vi "init.vi"(8 "error in":errorcluster, 10 "TBM module configuration in":refnum<class "TBM module configuration.lvclass">, 11 "Engine to Engine Communication runtime in":refnum<class "E2E Runtime (RT FIFO).lvclass">) -> (0 "error out":errorcluster, 1 "data allocations":T1, 2 "execution settings":T4, 3 "Engine to Engine Communication runtime out":refnum<class "E2E Runtime (RT FIFO).lvclass">)   [LabVIEW 2015, in "E2E Runtime (RT FIFO).lvclass"]
doc: "Provides an interface for initializing a module at runtime. While this interface performs no operations, a child should provide an override which may open any necessary references or sessions, allocate necessary memory, and perform any final configuration validataion before providing the full configuration <b>execution data</b> to the calling process."
uses:
  E2E Runtime (RT FIFO).lvclass
  <vilib>/NI/Tag Bus Module Framework/module configuration/TBM module configuration.lvclass
  <vilib>/NI/Tag Bus Module Framework/runtime/execution settings.ctl
  <vilib>/NI/Tag Bus Module Framework/channel/data tables.ctl
  <vilib>/NI/Tag Bus/dictionary/data dictionary.lvclass
  <vilib>/NI/Tag Bus/dictionary table pair.ctl
  <vilib>/NI/Tag Bus/table/data table.ctl
  configuration/E2E Tag Exchange configuration.lvclass
  <vilib>/NI/Configuration Framework/serializable configuration/NISE_CEF_serializable configuration.lvclass/NISE_CEF_serializable configuration.ctl
  configuration/E2E Tag Exchange configuration.lvclass/E2E Tag Exchange configuration.ctl
  E2E Runtime (RT FIFO).lvclass/E2E Runtime (RT FIFO).ctl
  <vilib>/Utility/LVClass/Get LV Class Name.vi
  <vilib>/NI/Configuration Framework/error generator/NISE_error generator.vi
  <vilib>/NI/Tag Bus Module Framework/channel/TBM channel.lvclass
  <vilib>/NI/Tag Bus Module Framework/runtime/TBM module execution interface.lvclass
  <vilib>/NI/Configuration Framework/serializable configuration/NISE_CEF_serializable configuration.lvclass
  <vilib>/NI/Tag Bus/tag bus.lvlib
  <vilib>/NI/Tag Bus/table/data table.lvlib
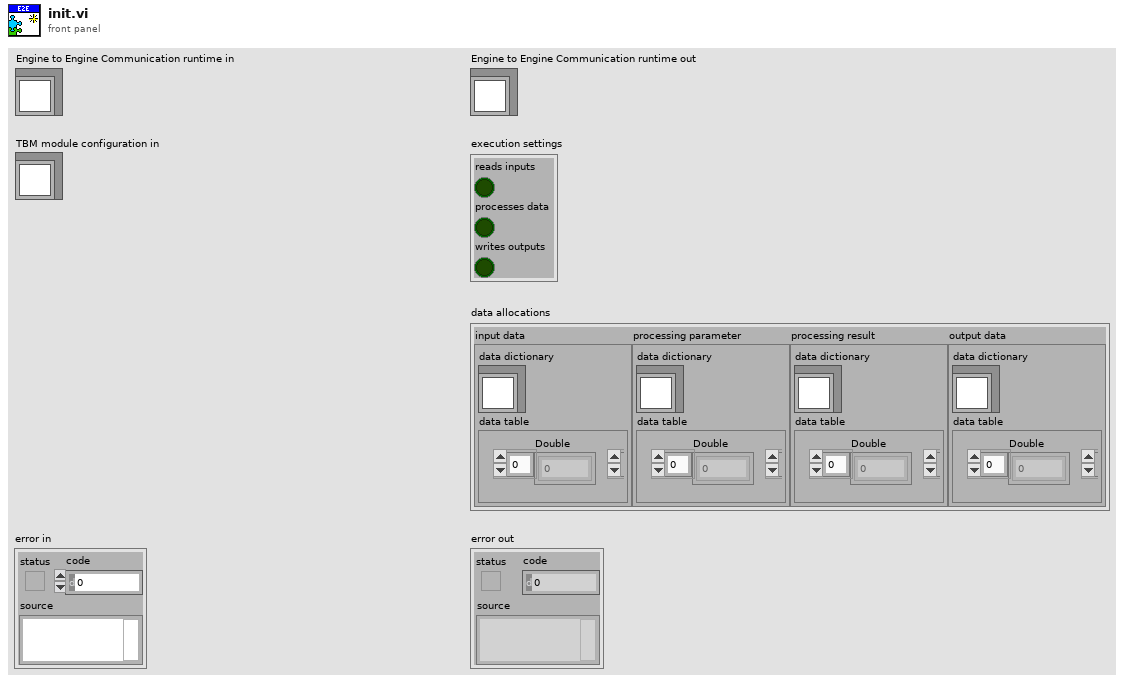
[diagram p1: front panel]
types:
  T1 = typedef "TBM channel.lvclass/data tables.ctl" = cluster{"input data":T2, "processing parameter":T2, "processing result":T2, "output data":T2}
  T2 = typedef "tag bus.lvlib/dictionary table pair.ctl" = cluster{"data dictionary":refnum<class "data dictionary.lvclass">, "data table":T3}
  T3 = typedef "tag bus.lvlib/data table.lvlib/data table.ctl" = cluster{"Double":dbl[], "Single":sgl[], "I64":i64[], "I32":i32[], "I16":i16[], "I8":i8[], "U64":u64[], "U32":u32[], "U16":u16[], "U8":u8[], "Boolean":bool[], "String":string[], "Array of Double":cluster{"DBL Array":dbl[]}[], "Array of Single":cluster{"SGL Array":sgl[]}[], "Array of I64":cluster{"I64 Array":i64[]}[], "Array of I32":cluster{"I32 Array":i32[]}[], "Array of I16":cluster{"I16 Array":i16[]}[], "Array of I8":cluster{"I8 Array":i8[]}[], "Array of U64":cluster{"U64 Array":u64[]}[], "Array of U32":cluster{"U32 Array":u32[]}[], "Array of U16":cluster{"U16 Array":u16[]}[], "Array of U8":cluster{"U8 Array":u8[]}[], "Array of Boolean":cluster{"Boolean Array":bool[]}[], "Array of String":cluster{"String Array":string[]}[]}
  T4 = typedef "TBM module execution interface.lvclass/execution settings.ctl" = cluster{"reads inputs":bool, "processes data":bool, "writes outputs":bool}
  T5 = typedef "tag bus.lvlib/data table.lvlib/allocation specification.ctl" = cluster{"data type":T6, "size":i32}
  T6 = typedef "tag bus.lvlib/tag descriptor.lvclass/Data Type.ctl" = enum16{"Double", "Single", "I64", "I32", "I16", "I8", "U64", "U32", "U16", "U8", "Boolean", "String", "Array of Double", "Array of Single", "Array of I64", "Array of I32", "Array of I16", "Array of I8", "Array of U64", "Array of U32", "Array of U16", "Array of U8", "Array of Boolean", "Array of String"}
  T7 = typedef "E2E Runtime (RT FIFO).lvclass/Data FIFOs.ctl" = cluster{"Double":refnum<k33>, "Single":refnum<k33>, "I64":refnum<k33>, "I32":refnum<k33>, "I16":refnum<k33>, "I8":refnum<k33>, "U64":refnum<k33>, "U32":refnum<k33>, "U16":refnum<k33>, "U8":refnum<k33>, "Boolean":refnum<k33>}
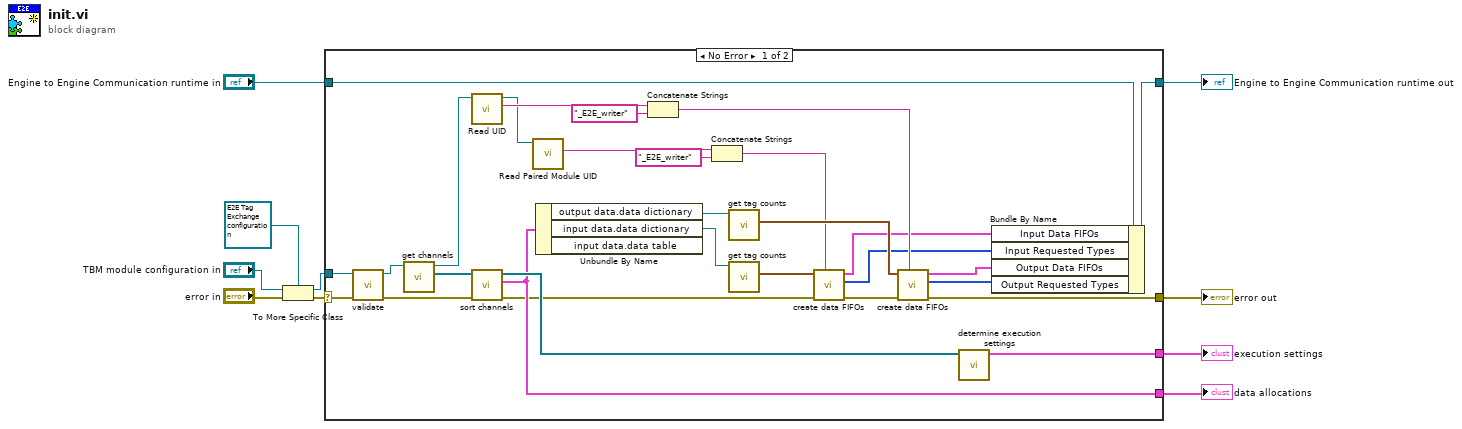
[diagram p0: block diagram]
diagram:
  n1 = To More Specific Class(target class=refnum<class "E2E Tag Exchange configuration.lvclass"> refnum ("E2E configuration"), reference="TBM module configuration in", error in="error in") -> (specific class reference=w9:refnum<class "E2E Tag Exchange configuration.lvclass">, error out=w10:errorcluster)
  n2 = case shown="No Error" w10 {
    selector: w10 -> [w36 w40]
    tunnel: w9 -> [w35 _]
    tunnel: "Engine to Engine Communication runtime in" -> [w19 w41]
    tunnel: [w18 w41] -> w5
    tunnel: [w24 w40] -> w4
    tunnel: [w32 _] -> w2
    tunnel: [w39 _] -> w3
    frame No Error {
      n3 = call-dynamic "validate.vi"("error in"=w36, "E2E Tag Exchange configuration in"=w35) -> ("error out"=w37:errorcluster, "E2E Tag Exchange configuration out"=w34:refnum<class "E2E Tag Exchange configuration.lvclass">)  [unwired: 8 in]
      n4 = call-dynamic "get channels.vi"("E2E configuration in"=w34) -> ("channels"=w33:refnum<class "TBM channel.lvclass">[], "E2E configuration out"=w30:refnum<class "E2E Tag Exchange configuration.lvclass">)  [unwired: 9 in]
      n5 = call <vilib>:"Read UID.vi"("configuration in"=w30) -> ("instance id"=w13:string, "configuration out"=w12:refnum<class "E2E Tag Exchange configuration.lvclass">)  [unwired: 8 in, 1 out]
      n6 = call <vilib>:"sort channels.vi"("error in"=w37, "channels in"=w33) -> ("error out"=w28:errorcluster, "data allocations"=w32:T1, "channels out"=w38:refnum<class "TBM channel.lvclass">[])  [unwired: 7 in]
      n7 = call "Read Paired Module UID.vi"("E2E Tag Exchange configuration in"=w12) -> ("Paired Module UID"=w11:string)  [unwired: 8 in, 2 out]
      n8 = Unbundle By Name(w32) -> ("output data.data dictionary"=w27:refnum<class "data dictionary.lvclass">, "input data.data dictionary"=w31:refnum<class "data dictionary.lvclass">)  [unwired: 1 out]
      n9 = Concatenate Strings(w13, "_E2E_writer" ("string")) -> (w21:string)
      n10 = Concatenate Strings(w11, "_E2E_writer" ("string")) -> (w20:string)
      n11 = call <vilib>:"get tag counts.vi"("data dictionary in"=w27) -> ("counts"=w25:T5[])  [unwired: 9 in, 1 out]
      n12 = call <vilib>:"get tag counts.vi"("data dictionary in"=w31) -> ("counts"=w29:T5[])  [unwired: 9 in, 1 out]
      n13 = call "create data FIFOs.vi"("FIFO name prefix"=w20, "error in (no error)"=w28, "counts"=w29) -> ("error out"=w26:errorcluster, "Requested Types"=w14:T6[], "Data FIFOs"=w17:T7)  [unwired: 6 in]
      n14 = call "create data FIFOs.vi"("FIFO name prefix"=w21, "error in (no error)"=w26, "counts"=w25) -> ("error out"=w24:errorcluster, "Requested Types"=w15:T6[], "Data FIFOs"=w16:T7)  [unwired: 6 in]
      n15 = call <vilib>:"determine execution settings.vi"("channels"=w38) -> ("execution settings"=w39:T4)  [unwired: 10 in]
      n16 = Bundle By Name(cluster=w19, "Input Data FIFOs"=w17, "Input Requested Types"=w14, "Output Data FIFOs"=w16, "Output Requested Types"=w15) -> (w18:refnum<class "E2E Runtime (RT FIFO).lvclass">)
    }
    frame Error {
    }
  }
  "error out" <- w4
  "Engine to Engine Communication runtime out" <- w5
  "execution settings" <- w3
  "data allocations" <- w2
